vi "Stop All.vi"(8 "Error in":errorcluster, 9 "Stop Configuration (All)":T1={"Stop the monitor? (true)"=TRUE, "Stop the remote terminals? (true)"=TRUE, "Stop the bus controller? (true)"=TRUE}, 11 "Module Handle out":u32) -> (0 "Error Out":errorcluster, 3 "Module Handle out":u32)   [LabVIEW 2020, in "AIM MIL-STD-1553 Hardware API.lvlib"]
doc: "<B>Input Parameters:</B>\n\nModule Handle - Reference to the device as obtained from a call to: 1553 General - Obtain a Device Reference.vi\n\nBIU Number (1) - BIU number (one-based) of the bus interface unit.\n\n<B> Output Parameters: </B>"
uses:
  AIM MIL-STD-1553 Hardware API.lvlib
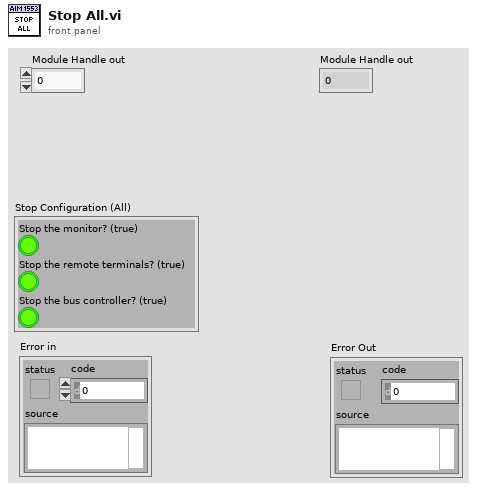
[diagram p1: front panel]
types:
  T1 = cluster{"Stop the monitor? (true)":bool, "Stop the remote terminals? (true)":bool, "Stop the bus controller? (true)":bool}
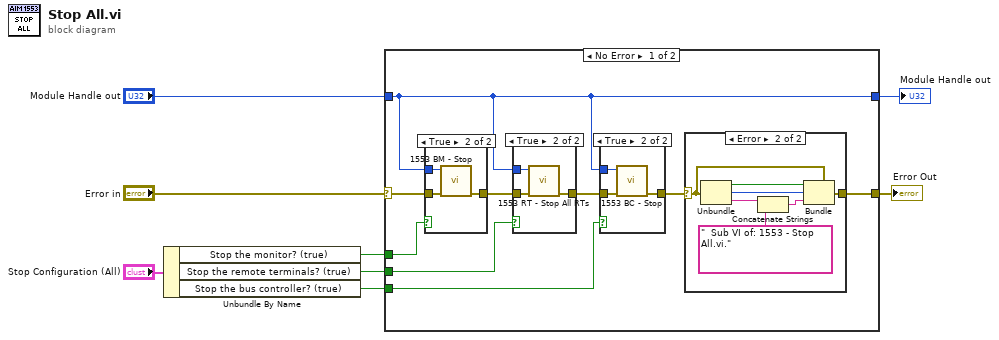
[diagram p0: block diagram]
diagram:
  n1 = Unbundle By Name("Stop Configuration (All)") -> ("Stop the monitor? (true)"=w5:bool, "Stop the remote terminals? (true)"=w4:bool, "Stop the bus controller? (true)"=w3:bool)
  n2 = case shown="No Error" "Error in" {
    selector: "Error in" -> [w17 w39]
    tunnel: [w13 w39] -> w7
    tunnel: "Module Handle out" -> [w9 w38]
    tunnel: w5 -> [w12 _]
    tunnel: w4 -> [w11 _]
    tunnel: w3 -> [w10 _]
    tunnel: [w9 w38] -> w1
    frame No Error {
      n3 = case shown="True" w12 {
        tunnel: w17 -> [w34 w37]
        tunnel: [w34 w36] -> w16
        tunnel: w9 -> [_ w35]
        frame False {
        }
        frame True {
          n4 = call <instrlib>:"1553 BM - Stop.vi"("Error In (none)"=w37, "Module Handle"=w35) -> ("Error Out"=w36:errorcluster)  [unwired: 8 in, 1 out]
        }
      }
      n5 = case shown="True" w11 {
        tunnel: w16 -> [w30 w33]
        tunnel: [w30 w32] -> w15
        tunnel: w9 -> [_ w31]
        frame False {
        }
        frame True {
          n6 = call <instrlib>:"1553 RT - Stop All RTs.vi"("Error In (none)"=w33, "Module Handle"=w31) -> ("Error Out"=w32:errorcluster)  [unwired: 8 in, 1 out]
        }
      }
      n7 = case shown="True" w10 {
        tunnel: w15 -> [w18 w21]
        tunnel: w9 -> [_ w20]
        tunnel: [w18 w19] -> w14
        frame False {
        }
        frame True {
          n8 = call <instrlib>:"1553 BC - Stop.vi"("Error In (none)"=w21, "Module Handle"=w20) -> ("Error Out"=w19:errorcluster)  [unwired: 8 in, 1 out]
        }
      }
      n9 = case shown="Error" w14 {
        selector: w14 -> [w22 w29]
        tunnel: [w22 w26] -> w13
        frame No Error {
        }
        frame Error {
          n10 = Unbundle(w29) -> ("status"=w27:bool, "code"=w28:i32, "source"=w25:string)
          n11 = Concatenate Strings(w25, "  Sub VI of: 1553 - Stop All.vi.") -> (w24:string)
          n12 = Bundle(cluster=w29, "status"=w27, "code"=w28, "source"=w24) -> (w26:errorcluster)
        }
      }
    }
    frame Error {
    }
  }
  "Error Out" <- w7
  "Module Handle out" <- w1
